vi "Scalar.vi"(2 "Scalar":dbl, 3 "Joystick Value":dbl) -> (1 "Final Joystick Value":dbl)   [LabVIEW 2020]
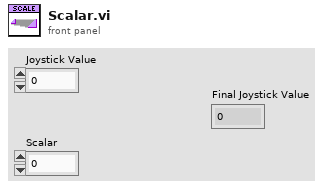
[diagram p1: front panel]
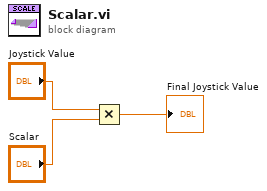
[diagram p0: block diagram]
diagram:
  n1 = Multiply(x="Joystick Value", y="Scalar") -> (x*y=→"Final Joystick Value":dbl)
